vi "Program File Call.vi"(11 "File path":path) -> (3 "Output":string[](array[string]))   [LabVIEW 2015]
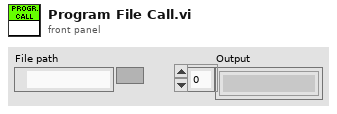
[diagram p1: front panel]
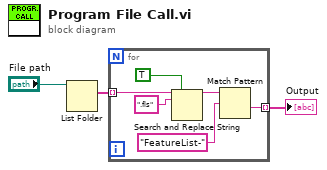
[diagram p0: block diagram]
diagram:
  n1 = List Folder(path="File path") -> (filenames=w1:string[])  [unwired: 3 in, 3 out]
  n2 = for {
    tunnel: w1 -> [w9] mode=indexing
    tunnel: [w4] -> w2 mode=indexing
    n3 = Search and Replace String(replace all?=TRUE ("replace all? (F)"), input string=w9, search string=".fls") -> (result string=w5:string)  [unwired: 5 in, 3 out]
    n4 = Match Pattern(string=w5, regular expression="FeatureList-") -> (after substring=w4:string)  [unwired: 1 in, 3 out]
  }
  "Output" <- w2
